vi "rc_initialize imu.vi"(6 "error in (no error)":errorcluster, 8 "Cluster":T1={"accel_fsr"=0, "gyro_fsr"=0, "gyro_dlpf"=0, "accel_dlpf"=0, "enable_magnetometer"=0, "dmp_sample_rate"=0, "orientation"=136, "compass_mix_factor"=0, "dmp_interrupt_priority"=0, "show_warnings"=0} {"orientation" items=["ORIENTATION_Z_UP"=136, "ORIENTATION_Z_DOWN"=396, "ORIENTATION_X_UP"=14, "ORIENTATION_X_DOWN"=266, "ORIENTATION_Y_UP"=112, "ORIENTATION_Y_DOWN"=336]; "accel_dlpf" items=["ACCEL_DLPF_OFF", "ACCEL_DLPF_184", "ACCEL_DLPF_92", "ACCEL_DLPF_41", "ACCEL_DLPF_20", "ACCEL_DLPF_10", "ACCEL_DLPF_5"]; "gyro_dlpf" items=["GYRO_DLPF_OFF", "GYRO_DLPF_184", "GYRO_DLPF_92", "GYRO_DLPF_41", "GYRO_DLPF_20", "GYRO_DLPF_10", "GYRO_DLPF_5"]; "gyro_fsr" items=["G_FSR_250DPS", "G_FSR_500DPS", "G_FSR_1000DPS", "G_FSR_2000DPS"]; "accel_fsr" items=["A_FSR_2G", "A_FSR_4G", "A_FSR_8G", "A_FSR_16G"]}, 9 "data":T2) -> (0 "error out":errorcluster, 2 "function return":i32, 3 "data out":T2)   [LabVIEW 2014, in "libroboticscape.lvlib"]
doc: "int initialize_imu(imu_data_t *data, imu_config_t conf);"
uses:
  libroboticscape.lvlib
  controls/imu_config_t.ctl
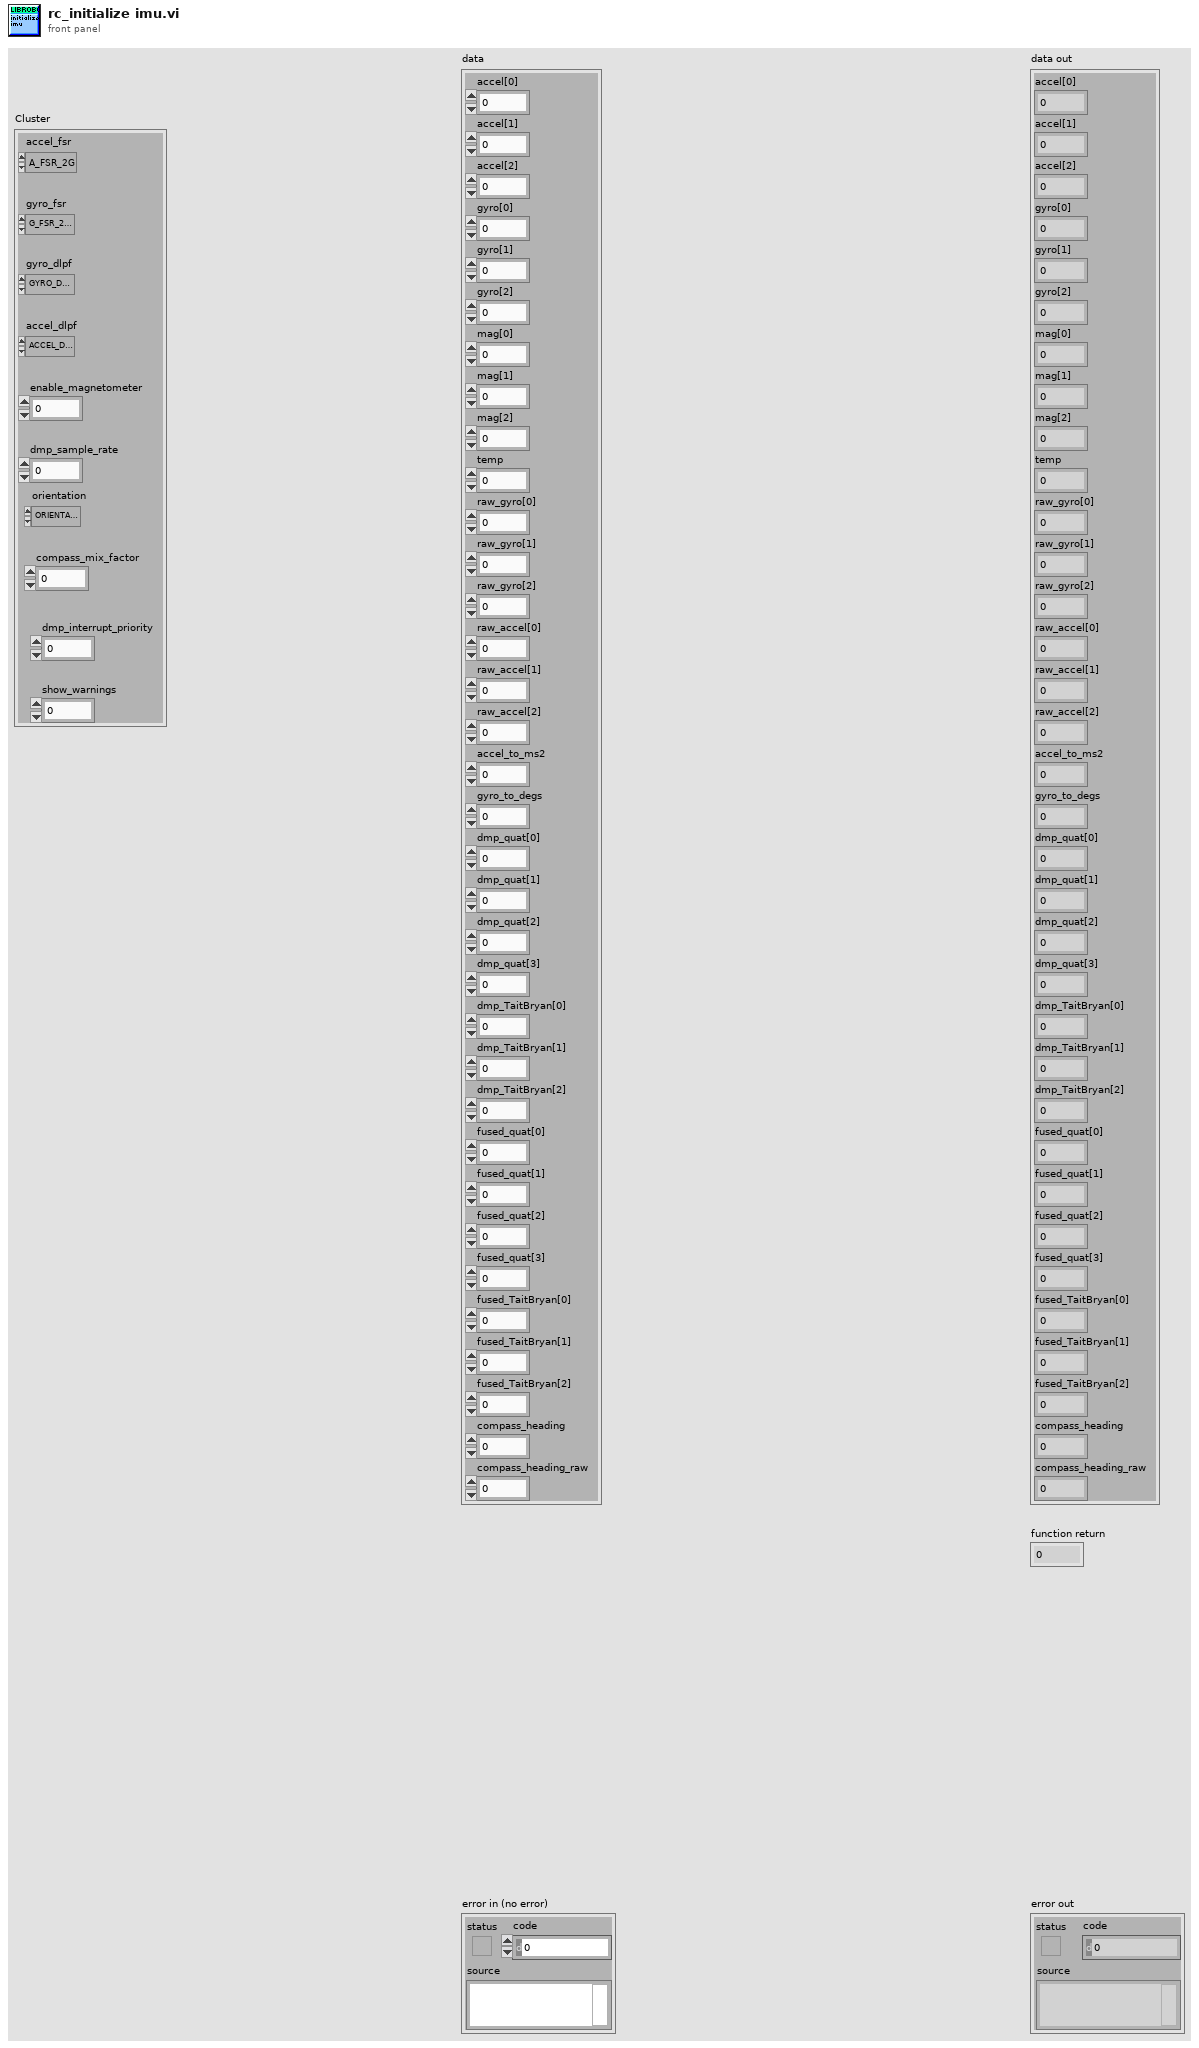
[diagram p1: front panel]
types:
  T1 = typedef "libroboticscape.lvlib/imu_config_t.ctl" = cluster{"accel_fsr":u32, "gyro_fsr":u32, "gyro_dlpf":u32, "accel_dlpf":u32, "enable_magnetometer":i32, "dmp_sample_rate":i32, "orientation":u32, "compass_mix_factor":i32, "dmp_interrupt_priority":i32, "show_warnings":i32}
  T2 = cluster{"accel[0]":sgl, "accel[1]":sgl, "accel[2]":sgl, "gyro[0]":sgl, "gyro[1]":sgl, "gyro[2]":sgl, "mag[0]":sgl, "mag[1]":sgl, "mag[2]":sgl, "temp":sgl, "raw_gyro[0]":i16, "raw_gyro[1]":i16, "raw_gyro[2]":i16, "raw_accel[0]":i16, "raw_accel[1]":i16, "raw_accel[2]":i16, "accel_to_ms2":sgl, "gyro_to_degs":sgl, "dmp_quat[0]":sgl, "dmp_quat[1]":sgl, "dmp_quat[2]":sgl, "dmp_quat[3]":sgl, "dmp_TaitBryan[0]":sgl, "dmp_TaitBryan[1]":sgl, "dmp_TaitBryan[2]":sgl, "fused_quat[0]":sgl, "fused_quat[1]":sgl, "fused_quat[2]":sgl, "fused_quat[3]":sgl, "fused_TaitBryan[0]":sgl, "fused_TaitBryan[1]":sgl, "fused_TaitBryan[2]":sgl, "compass_heading":sgl, "compass_heading_raw":sgl}
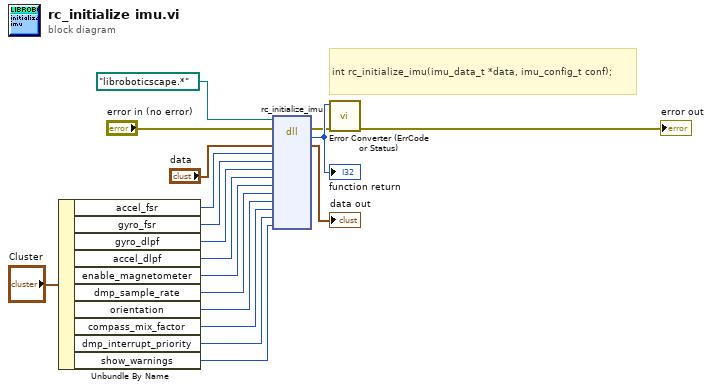
[diagram p0: block diagram]
diagram:
  # "int rc_initialize_imu(imu_data_t *data, imu_config_t conf);"
  n1 = Unbundle By Name("Cluster") -> ("accel_fsr"=w10:u32, "gyro_fsr"=w9:u32, "gyro_dlpf"=w8:u32, "accel_dlpf"=w7:u32, "enable_magnetometer"=w6:i32, "dmp_sample_rate"=w5:i32, "orientation"=w4:u32, "compass_mix_factor"=w3:i32, "dmp_interrupt_priority"=w2:i32, "show_warnings"=w1:i32)
  n2 = dll-call lib="C:/Users/ktalke/Documents/Robotics-Cape-Master-Jessie/Libroboticscape-Master-Jessie/libroboticscape.so" fn="rc_initialize_imu"(path in=path "libroboticscape.*", error in="error in (no error)", "data"="data", "accel_fsr"=w10, "gyro_fsr"=w9, "gyro_dlpf"=w8, "accel_dlpf"=w7, "enable_magnetometer"=w6, "dmp_sample_rate"=w5, "orientation"=w4, "compass_time_constant"=w3, "dmp_interrupt_priority"=w2, "show_warnings"=w1) -> (error out=w14:errorcluster, "return type"=w18:i32, "data"=→"data out":T2)  [unwired: 11 in, 1 out]
  "function return" <- w18
  n3 = call "Error Converter (ErrCode or Status).vi"("error in (no error)"=w14, "error code"=w18) -> ("error out"=→"error out":errorcluster)  [unwired: 9 in]
